vi "auto Set SR830 SENS (SubVI).vi"(8 "error in (no error)":errorcluster, 11 "VISA Refnum in":refnum<visa-resource-name>) -> (0 "error out":errorcluster, 3 "VISA Refnum out":refnum<visa-resource-name>)   [LabVIEW 2019, in "User lib.lvlib"]
uses:
  User lib.lvlib
  lib/Stanford Research 830/Public/Data/Read (1 Parameter).vi
  lib/Stanford Research 830/Stanford Research 830.lvlib
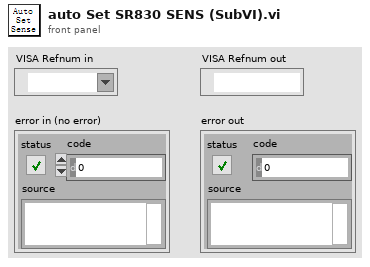
[diagram p1: front panel]
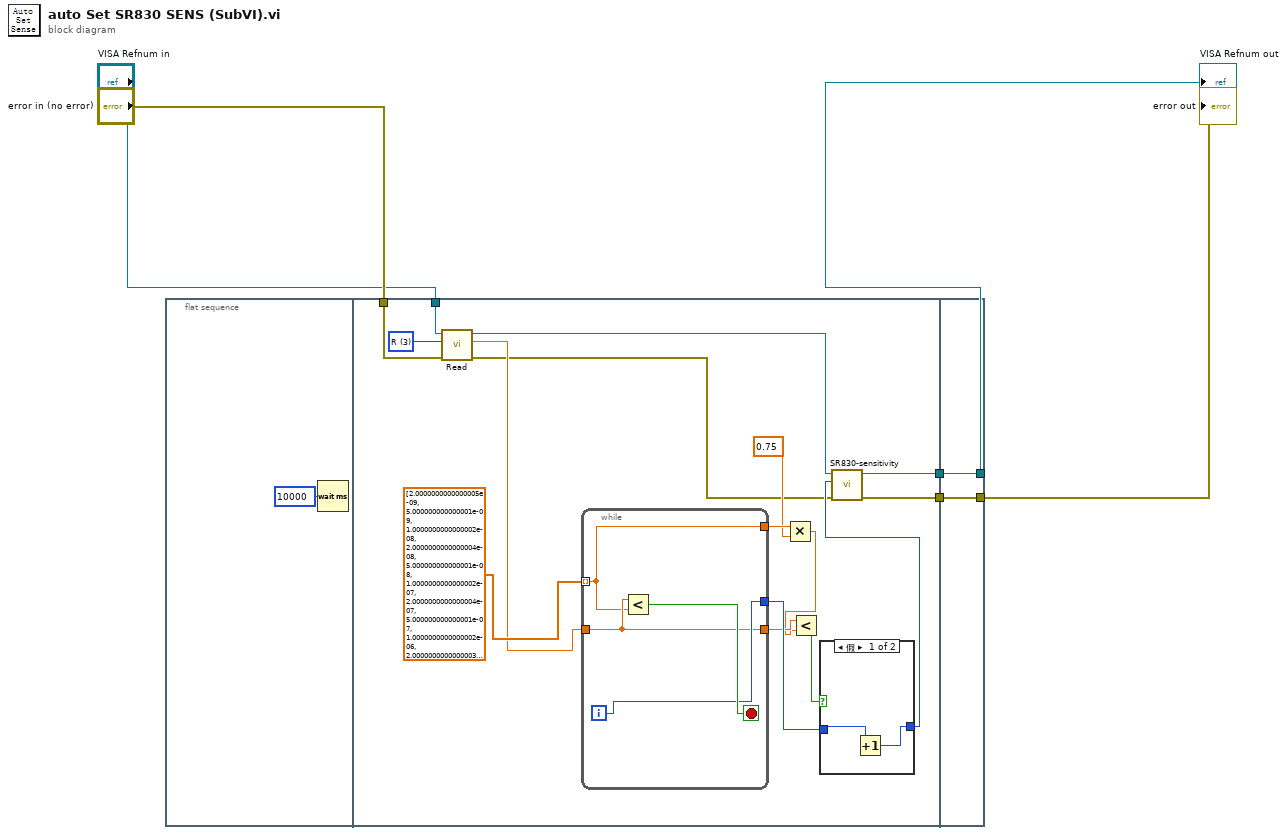
[diagram p0: block diagram]
diagram:
  n1 = flat-sequence {
    tunnel: "VISA Refnum in" -> [w19]
    tunnel: "error in (no error)" -> [w10]
    tunnel: [w18] -> w2
    tunnel: [w8] -> w1
    tunnel: [w31] -> w6
    tunnel: [w32] -> w4
    tunnel: w2 -> [w32]
    tunnel: w1 -> [w31]
    frame #0 {
      n2 = Wait (ms)(milliseconds to wait=u32 10000) -> ()  [unwired: 1 out]
    }
    frame #1 {
      w23 = u16 3 items=["X"=1, "Y"=2, "R"=3, "Theta"=4, "Channel 1"=5, "Channel 2"=6, "Aux In 1"=7, "Aux In 2"=8, "Aux In 3"=9, "Aux In 4"=10] ("Parameter (1: X)")
      n3 = call-poly "Read.vi"("error in (no error)"=w10, "Parameter (1: X)"=w23, "VISA resource name"=w19) -> ("error out"=w9:errorcluster, "Measurement"=w21:dbl, "VISA resource name out"=w20:refnum<visa-resource-name>)  [unwired: 6 in]
      n4 = while {
        tunnel: dbl[] [2.0000000000000005e-09, 5.000000000000001e-09, 1.0000000000000002e-08, 2.0000000000000004e-08, 5.000000000000001e-08, 1.0000000000000002e-07, 2.0000000000000004e-07, 5.000000000000001e-07, 1.0000000000000002e-06, 2.0000000000000003e-06, 5e-06, 1e-05, 2e-05, 5e-05, 0.0001, 0.0002, 0.0005, 0.001, 0.002, 0.005, 0.01, 0.02, 0.05, 0.1, 0.2, 0.5, 1.0] ("array") -> [w27] mode=indexing
        tunnel: w21 -> [w28]
        tunnel: [w29] -> w17
        tunnel: [w28] -> w16
        tunnel: [w27] -> w15
        i -> [w29]
        stop <- w30 stop-if-true
        n5 = Less?(x=w28, y=w27) -> (x < y?=w30:bool)
      }
      n6 = Multiply(x=w15, y=0.75) -> (x*y=w13:dbl)
      n7 = Less?(x=w16, y=w13) -> (x < y?=w12:bool)
      n8 = case shown="假" w12 {
        tunnel: w17 -> [w25 w26]
        tunnel: [w24 w26] -> w11
        frame False {
          n9 = Increment(x=w25) -> (x+1=w24:i32)
        }
        frame True {
        }
      }
      n10 = call "SR830-sensitivity.vi"("error in (no error)"=w9, "Sensitivity (-1: Auto gain)"=w11, "VISA resource name"=w20) -> ("error out"=w8:errorcluster, "VISA resource name out"=w18:refnum<visa-resource-name>)  [unwired: 7 in]
    }
    frame #2 {
    }
  }
  "error out" <- w6
  "VISA Refnum out" <- w4
